vi "Check_Traverse_move_Low_PN.vi"(0 "Current position":sgl[](array[numeric])=[0.0, 200.0, 40.0] format="%.2f", 1 "New Position":sgl[](array[numeric])=[0.0, 100.0, 40.0] format="%.2f", 3 "Model       Roll      Pitch       Yaw (deg)":sgl[](array[numeric]) format="%#.2f", 4 "Traverse Name":string) -> (5 "Error Comments":string, 6 "Collision":bool)   [LabVIEW 2016]
uses:
  Collision_Detection/Triangles/EnFlo specific/Traverse active parts.ctl
  Collision_Detection/Triangles/EnFlo specific/Collision Mode.ctl
  Route_mapping_global.vi
  Collision_Detection/Triangles/EnFlo specific/Collision Detection global.vi
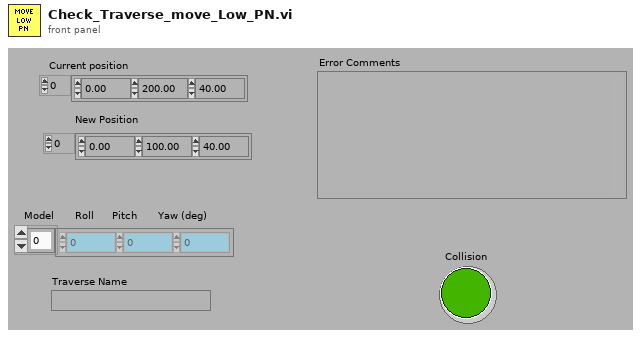
[diagram p1: front panel]
types:
  T1 = typedef "Box_size.ctl" = cluster{"Max":sgl, "Min":sgl}[]
  T2 = typedef "Traverse active parts.ctl" = enum16{"XYZ", "XY and XYZ", "X and XY and XYZ"}
  T3 = typedef "Collision Mode.ctl" = enum16{"Traverse - Tunnel", "Traverse - Model", "Traverse - Fixed objects", "Traverse - Traverse", "Traverse - All"}
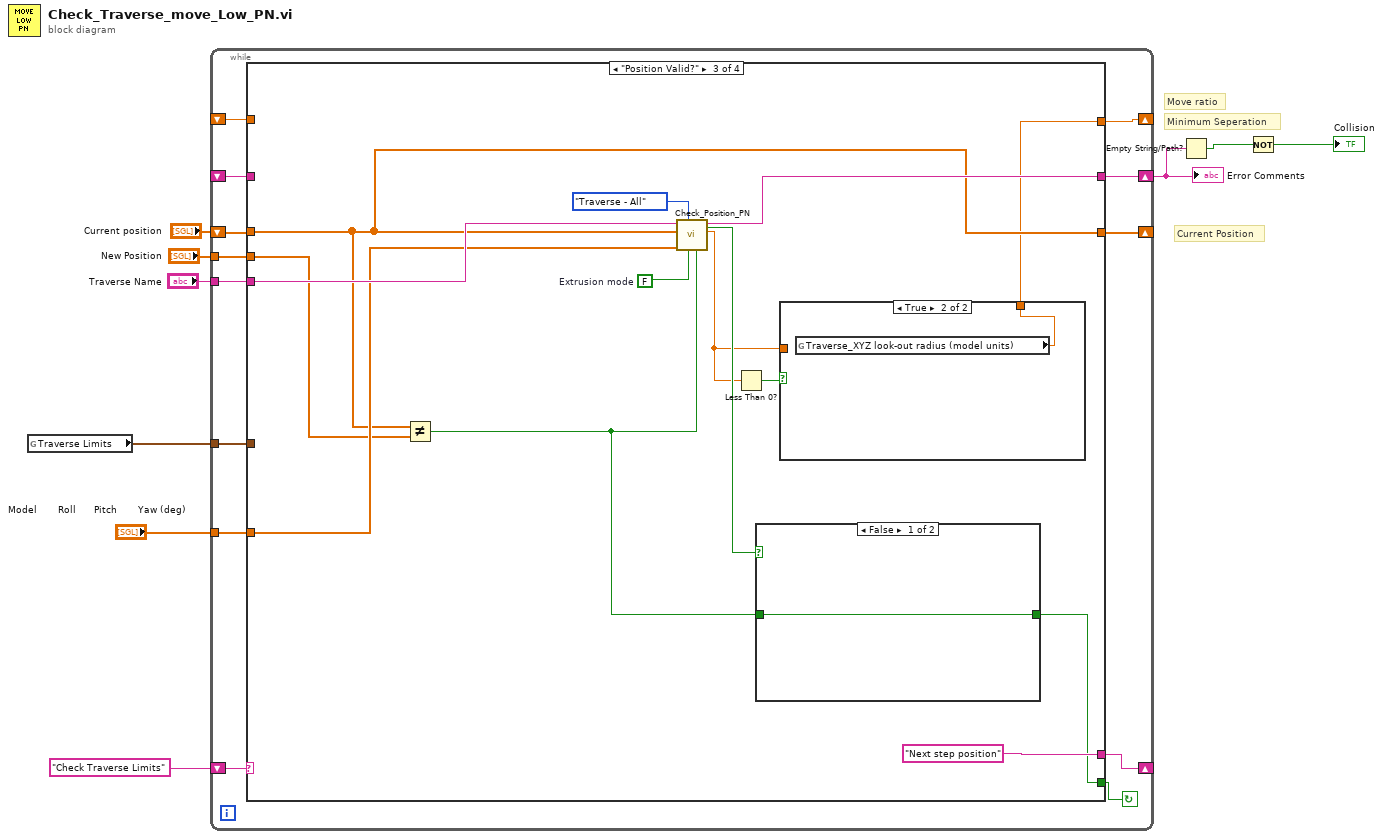
[diagram p0: block diagram]
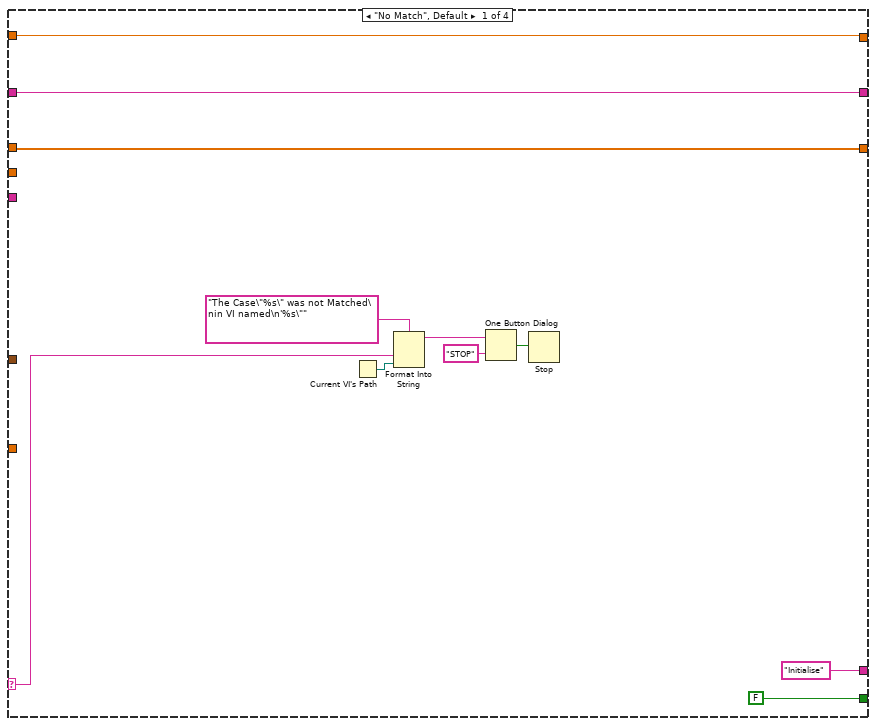
[diagram p2: hidden frame]
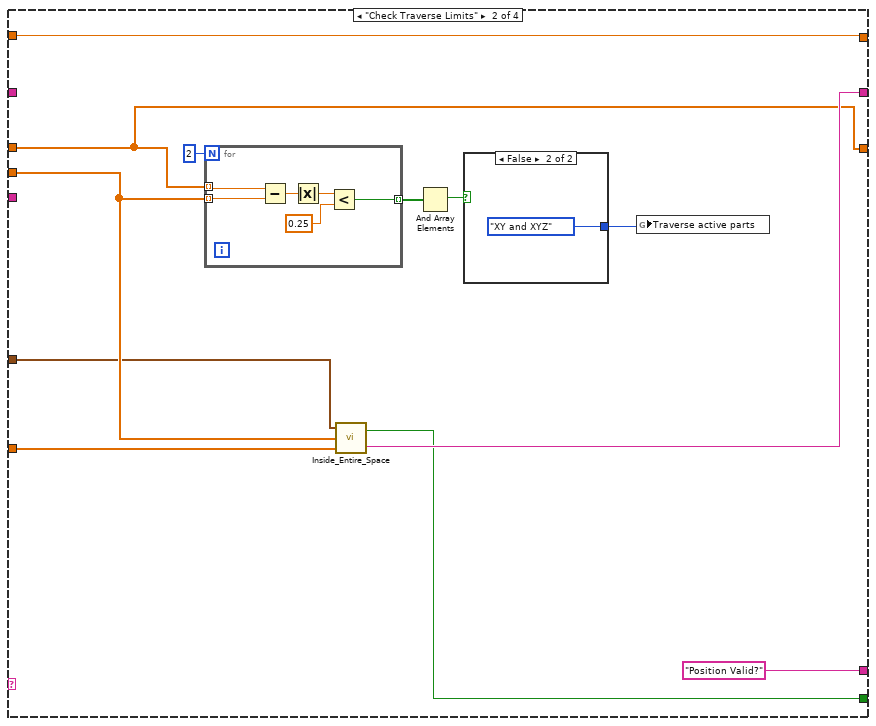
[diagram p3: hidden frame]
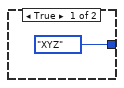
[diagram p4: hidden frame]
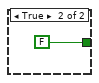
[diagram p6: hidden frame]
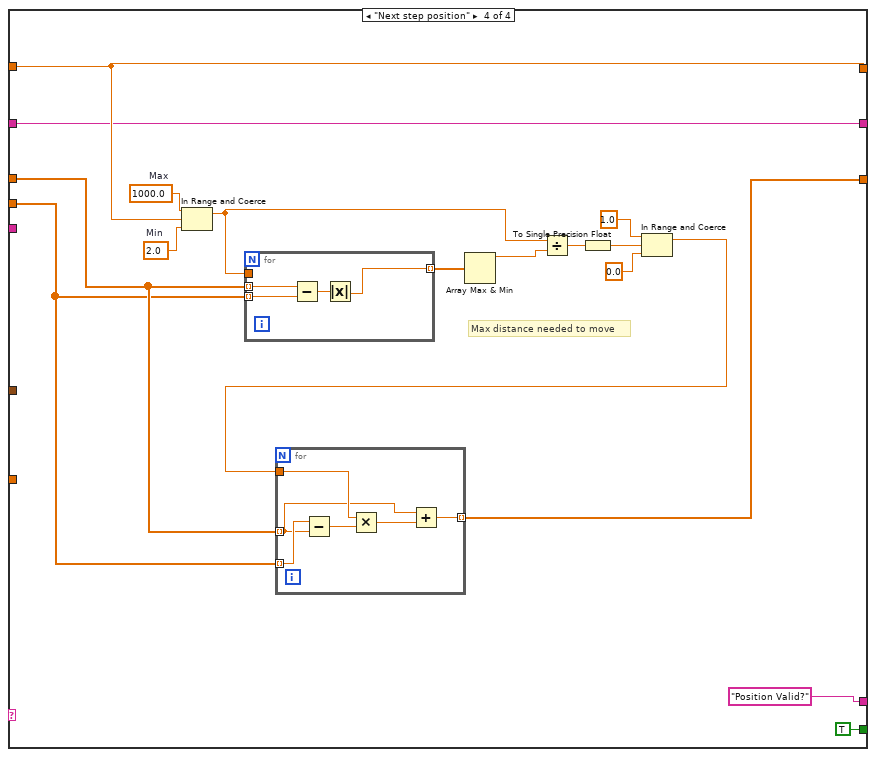
[diagram p7: hidden frame]
diagram:
  # "Current Position"
  # "Move ratio"
  # "Minimum Seperation"
  n1 = global read "Route_mapping_global.vi" "Traverse Limits"() -> (w6:T1)
  n2 = while {
    shift-left: "Check Traverse Limits" -> [w15]
    shift-right: [w22] -> _
    shift-right: [w19] -> w3
    shift-left: _ -> [w20]
    tunnel: "New Position" -> [w18]
    tunnel: "Traverse Name" -> [w17]
    tunnel: "Model       Roll      Pitch       Yaw (deg)" -> [w16]
    tunnel: w6 -> [w14]
    shift-right: [w13] -> _
    shift-left: _ -> [w12]
    shift-right: [w10] -> _
    shift-left: "Current position" -> [w11]
    stop <- w21 continue-if-true
    n3 = case shown="\"Position Valid?\"" w15 {
      selector: w15 -> [w25 _ _ _]
      tunnel: [FALSE w42 w62 TRUE ("Box Inside")] -> w21
      tunnel: ["Initialise" "Position Valid?" "Next step position" "Position Valid?"] -> w22
      tunnel: w20 -> [w26 _ _ w78]
      tunnel: [w26 w44 w64 w78] -> w19
      tunnel: w11 -> [w23 w34 w61 w81]
      tunnel: w18 -> [_ w40 w60 w80]
      tunnel: w17 -> [_ _ w66 _]
      tunnel: w16 -> [_ w45 w65 _]
      tunnel: w14 -> [_ w36 _ _]
      tunnel: [w24 w35 w55 w83] -> w13
      tunnel: w12 -> [w24 w35 _ w83]
      tunnel: [w23 w34 w61 w79] -> w10
      frame "No Match", Default {
        n4 = Current VI's Path() -> (path=w28:path)
        n5 = Format Into String(format string="The Case\"%s\" was not Matched\nin VI named\n'%s\"" ("Format String"), w25, w28) -> (resulting string=w31:string)  [unwired: 2 in, 1 out]
        n6 = One Button Dialog(message=w31, button name ("OK")="STOP") -> (true=w29:bool)
        n7 = Stop(stop? (T)=w29) -> ()
      }
      frame "Check Traverse Limits" {
        n8 = for {
          N: 2 -> [_]
          tunnel: w34 -> [w52] mode=indexing
          tunnel: w40 -> [w53] mode=indexing
          tunnel: [w48] -> w39 mode=indexing
          n9 = Subtract(x=w52, y=w53) -> (x-y=w51:sgl)
          n10 = Absolute Value(x=w51) -> (abs(x)=w50:sgl)
          n11 = Less?(x=w50, y=sgl 0.25) -> (x < y?=w48:bool)
        }
        n12 = call "Inside_Entire_Space.vi"("Model       Roll      Pitch       Yaw (deg)"=w45, "Current Position"=w40, "Envelope"=w36) -> ("Error Comments"=w44:string, "Box Inside"=w42:bool)
        n13 = And Array Elements(Boolean array=w39) -> (logical AND=w38:bool)
        n14 = case shown="False" w38 {
          tunnel: [Traverse_active_parts."XYZ" ("Traverse active parts") Traverse_active_parts."XY and XYZ" ("Traverse active parts")] -> w37
          frame True {
          }
          frame False {
          }
        }
        n15 = global write "Collision Detection global.vi" "Traverse active parts"(w37) -> ()
      }
      frame "Position Valid?" {
        w57 = FALSE  # Extrusion mode
        n16 = Not Equal?(x=w61, y=w60) -> (x != y?=w59:bool)
        n17 = call "Check_Position_PN.vi"("Get minimum separation within look-out sphere"=w59, "Extrusion mode"=w57, "Collision mode"=Collision_Mode."Traverse - All", "Model Rotation (deg)"=w65, "Position to check"=w61, "Traverse Name"=w66) -> ("Minimum separation"=w54:sgl, "Error Comments"=w64:string, "Collision"=w63:bool)  [unwired: 2 in, 1 out]
        n18 = Less Than 0?(x=w54) -> (x < 0?=w56:bool)
        n19 = case shown="False" w63 {
          tunnel: [w70 FALSE] -> w62
          tunnel: w59 -> [w70 _]
          frame False {
          }
          frame True {
          }
        }
        n20 = case shown="True" w56 {
          tunnel: [w68 w69] -> w55
          tunnel: w54 -> [w68 _]
          frame False {
          }
          frame True {
            n21 = global read "Collision Detection global.vi" "Traverse_XYZ look-out radius (model units)"() -> (w69:sgl)
          }
        }
      }
      frame "Next step position" {
        w85 = 1000.0  # Max
        w84 = 2.0  # Min
        # "Max distance needed to move"
        n22 = In Range and Coerce(upper limit=w85, x=w83, lower limit=w84) -> (coerced(x)=w88:dbl)  [unwired: 1 out]
        n23 = for {
          tunnel: w81 -> [w98] mode=indexing
          tunnel: w80 -> [w97] mode=indexing
          tunnel: w88 -> [_]
          tunnel: [w95] -> w86 mode=indexing
          n24 = Subtract(x=w98, y=w97) -> (x-y=w96:sgl)
          n25 = Absolute Value(x=w96) -> (abs(x)=w95:sgl)
        }
        n26 = Array Max & Min(array=w86) -> (max value=w87:sgl)  [unwired: 3 out]
        n27 = Divide(x=w88, y=w87) -> (x/y=w82:dbl)
        n28 = To Single Precision Float(number=w82) -> (single precision float=w75:sgl)
        n29 = In Range and Coerce(upper limit=sgl 1.0, x=w75, lower limit=sgl 0.0) -> (coerced(x)=w72:sgl)  [unwired: 1 out]
        n30 = for {
          tunnel: w80 -> [w94] mode=indexing
          tunnel: w81 -> [w90] mode=indexing
          tunnel: w72 -> [w92]
          tunnel: [w89] -> w79 mode=indexing
          n31 = Subtract(x=w94, y=w90) -> (x-y=w93:sgl)
          n32 = Multiply(x=w92, y=w93) -> (x*y=w91:sgl)
          n33 = Add(x=w90, y=w91) -> (x+y=w89:sgl)
        }
      }
    }
  }
  "Error Comments" <- w3
  n34 = Empty String/Path?(string/path=w3) -> (empty?=w2:bool)
  n35 = Not(x=w2) -> (.not. x?=→"Collision":bool)
